vi "RT_AMC_Main.vi"() -> ()   [LabVIEW 2010]
panel:
  out "Process":bool
  out "Status":string
  in  "State Variables":cluster{"CurrentFile":path}
  # "Target2"
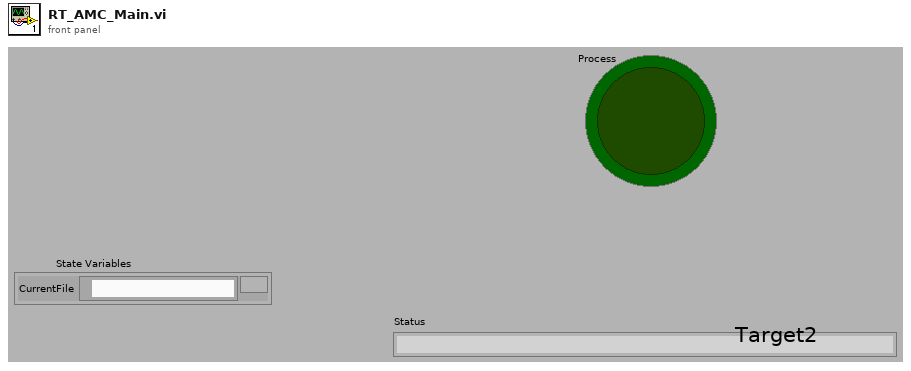
[diagram p1: front panel]
types:
  T1 = typedef "amc_Message Queue.ctl" = refnum<queue>
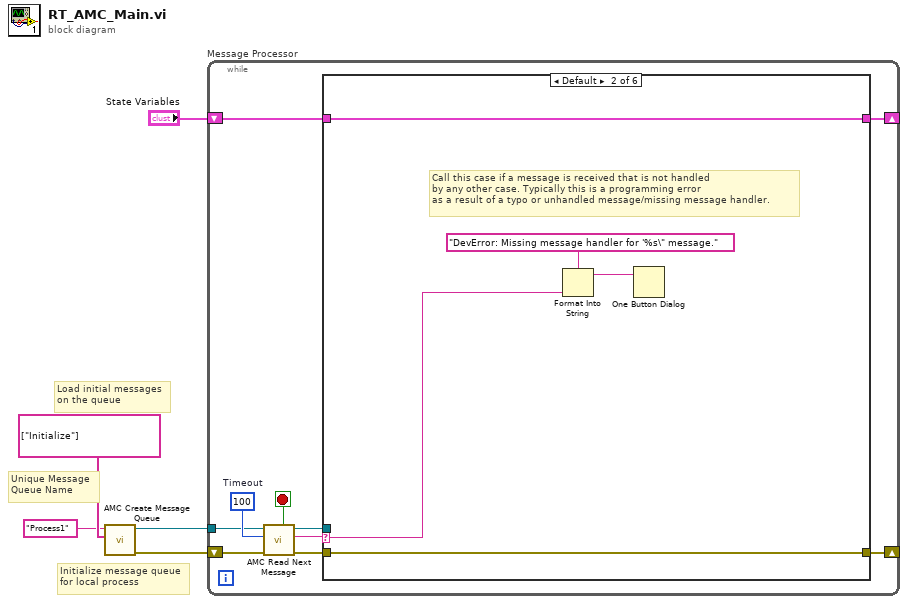
[diagram p0: block diagram]
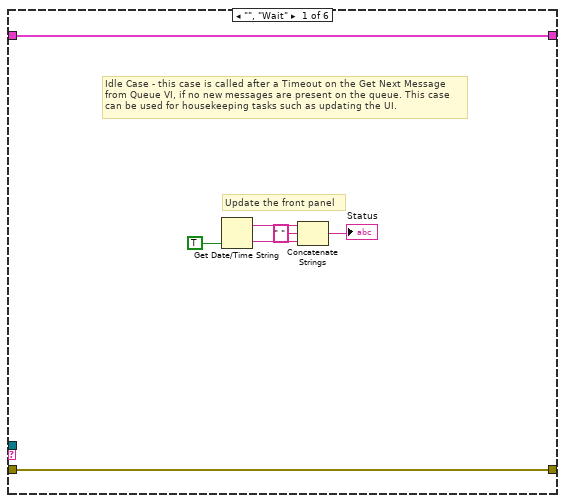
[diagram p2: hidden frame]
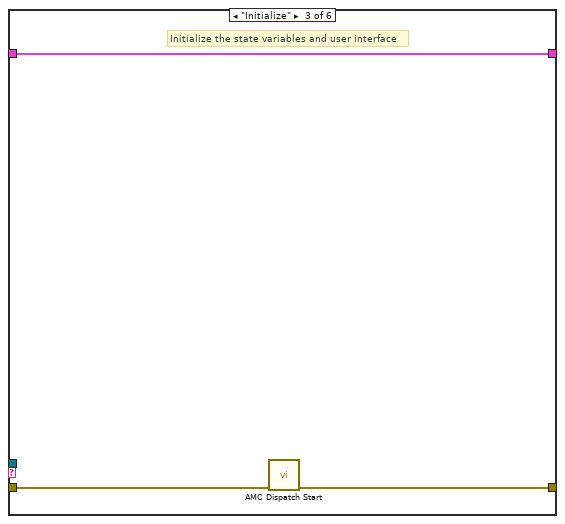
[diagram p3: hidden frame]
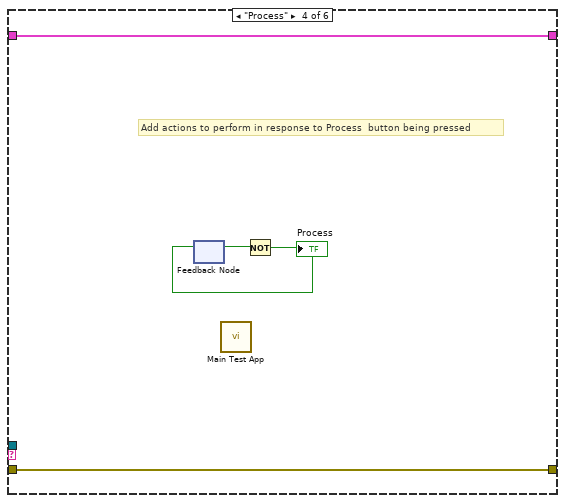
[diagram p4: hidden frame]
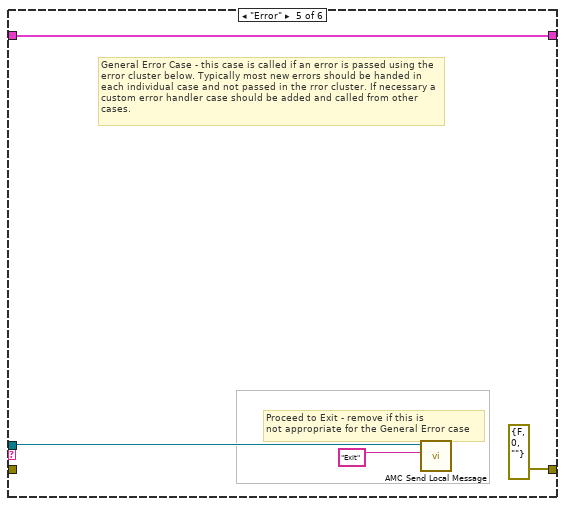
[diagram p5: hidden frame]
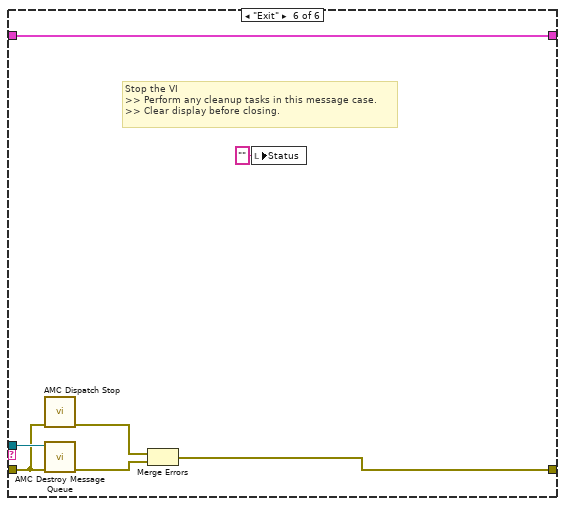
[diagram p6: hidden frame]
diagram:
  # "Initialize message queue\nfor local process"
  # "Unique Message\nQueue Name"
  # "Load initial messages\non the queue"
  n1 = call <userlib>:"AMC Create Message Queue.vi"("Initial Message Names"=string[] ["Initialize"], "Message Queue Name"="Process1" ("Message queue name (unnamed)")) -> ("error out"=w4:errorcluster, "Message Queue out"=w2:T1)  [unwired: 3 in, 5 out]
  n2 = while "Message Processor" {
    shift-left: w4 -> [w10]
    shift-right: [w11] -> _
    tunnel: w2 -> [w6]
    shift-left: "State Variables" -> [w15]
    shift-right: [w14] -> _
    stop <- w7 stop-if-true
    w9 = 100  # Timeout
    n3 = call <userlib>:"AMC Read Next Message.vi"("error in (no error)"=w10, "timeout (1ms)"=w9, "Message Queue in"=w6) -> ("error out"=w12:errorcluster, "Message Name"=w8:string, "Message Queue out"=w13:T1, "Exit Process"=w7:bool)  [unwired: 1 in, 4 out]
    n4 = case shown="Default" w8 {
      selector: w8 -> [_ w25 _ _ _ _]
      tunnel: [w22 w27 w30 w33 w38 w45] -> w14
      tunnel: w15 -> [w22 w27 w30 w33 w38 w45]
      tunnel: w13 -> [_ _ _ _ w36 w43]
      tunnel: w12 -> [w21 w26 w29 w34 _ w39]
      tunnel: [w21 w26 w28 w34 errorcluster {"status"=FALSE, "code"=0, "source"=""} ("error out") w40] -> w11
      frame "", "Wait" {
        # "Update the front panel"
        # "Idle Case - this case is called after a Timeout on the Get Next Message from Queue VI, if no new messages are present on the queue. This case can be used for housekeeping tasks such as updating the UI."
        n5 = Get Date/Time String(want seconds? (F)=TRUE) -> (date string=w20:string, time string=w19:string)  [unwired: 2 out]
        n6 = Concatenate Strings(w20, " " ("string"), w19) -> (→"Status":string)
      }
      frame Default {
        # "Call this case if a message is received that is not handled \nby any other case. Typically this is a programming error\nas a result of a typo or unhandled message/missing message handler."
        n7 = Format Into String(format string="DevError: Missing message handler for '%s\" message." ("message"), w25) -> (resulting string=w23:string)  [unwired: 2 in, 1 out]
        n8 = One Button Dialog(message=w23) -> ()  [unwired: 2 out]
      }
      frame "Initialize" {
        # "Initialize the state variables and user interface"
        n9 = call <userlib>:"AMC Dispatch Start.vi"("error in (no error)"=w29) -> ("error out"=w28:errorcluster)  [unwired: 1 in, 9 out]
      }
      frame "Process" {
        # "Add actions to perform in response to Process  button being pressed"
        n10 = feedback #1() -> (w32:bool)  [unwired: 1 out]
        n11 = call "Main Test App.vi"() -> ()  [unwired: 1 in]
        n12 = Not(x=w32) -> (.not. x?=w31:bool)
        "Process" <- w31
        n13 = feedback-in #1(w31) -> ()
      }
      frame "Error" {
        # "Proceed to Exit - remove if this is\nnot appropriate for the General Error case"
        # "General Error Case - this case is called if an error is passed using the error cluster below. Typically most new errors should be handed in each individual case and not passed in the rror cluster. If necessary a custom error handler case should be added and called from other cases."
        n14 = call <userlib>:"AMC Send Local Message.vi"("Message Name"="Exit", "Message Queue in"=w36) -> ()  [unwired: 4 in, 6 out]
      }
      frame "Exit" {
        # "Stop the VI\n>> Perform any cleanup tasks in this message case.\n>> Clear display before closing."
        n15 = call <userlib>:"AMC Dispatch Stop.vi"("error in (no error)"=w39) -> ("error out"=w41:errorcluster)  [unwired: 10 out]
        n16 = call <userlib>:"AMC Destroy Message Queue.vi"("error in (no error)"=w39, "Message Queue in"=w43) -> ("error out"=w42:errorcluster)  [unwired: 9 out]
        n17 = Merge Errors(w41, w42) -> (w40:errorcluster)
        n18 = local write "Status"("" ("Status")) -> ()
      }
    }
  }
